vi "Inspect row - one direction.vi"(10 "Trees in":T1[](array[typedef])) -> (2 "Trees out":T1[](array[typedef]))   [LabVIEW 2020]
uses:
  tree--cluster.ctl
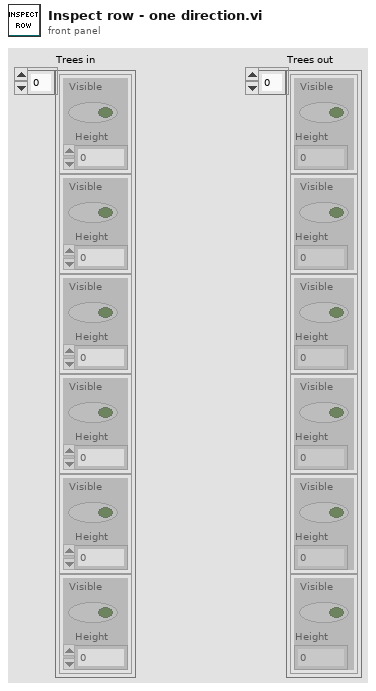
[diagram p1: front panel]
types:
  T1 = typedef "tree--cluster.ctl" = cluster{"Visible":bool, "Height":i32}
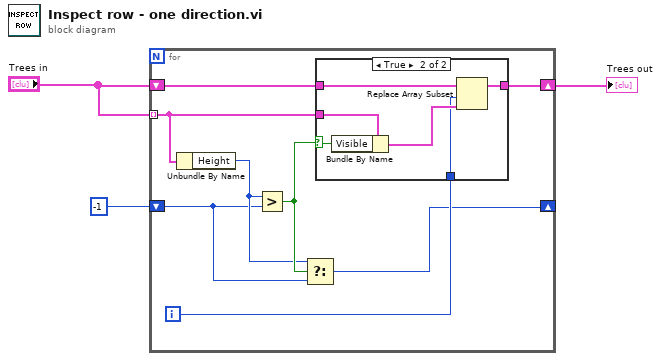
[diagram p0: block diagram]
diagram:
  n1 = for {
    tunnel: "Trees in" -> [w11] mode=indexing
    shift-right: [w4] -> _
    shift-left: -1 -> [w5]
    shift-right: [w10] -> w1
    shift-left: "Trees in" -> [w9]
    i -> [w8]
    n2 = Unbundle By Name(w11) -> ("Height"=w6:i32)
    n3 = Greater?(x=w6, y=w5) -> (0:w7:bool)
    n4 = Select(t=w6, s=w7, f=w5) -> (s? t:f=w4:i32)
    n5 = case shown="True" w7 {
      selector: w7 -> [_ w13]
      tunnel: w11 -> [_ w18]
      tunnel: [w12 w17] -> w10
      tunnel: w9 -> [w12 w16]
      tunnel: w8 -> [_ w14]
      frame False {
      }
      frame True {
        n6 = Bundle By Name(cluster=w18, "Visible"=w13) -> (w15:T1)
        n7 = Replace Array Subset(array=w16, new element=w15, index=w14) -> (w17:T1[])
      }
    }
  }
  "Trees out" <- w1
